vi "Log Error.vi"(8 "Error In":errorcluster, 10 "Error To Log":errorcluster, 11 "Error Handling In":refnum<class "Error Handling.lvclass">) -> (0 "Error Out":errorcluster, 3 "Error Handling Out":refnum<class "Error Handling.lvclass">)   [LabVIEW 2021, in "Error Handling.lvclass"]
uses:
  Error Handling.lvclass
  Accessors/Log File Reference/Get Log File Reference.vi
  Accessors/Log File Reference/Set Log File Reference.vi
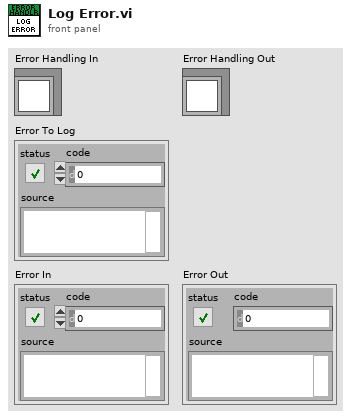
[diagram p1: front panel]
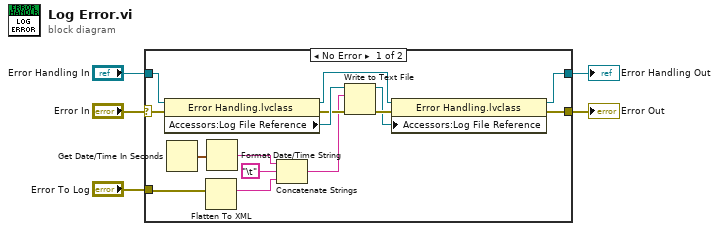
[diagram p0: block diagram]
diagram:
  n1 = case shown="No Error" "Error In" {
    selector: "Error In" -> [w20 w21]
    tunnel: "Error Handling In" -> [w19 w22]
    tunnel: [w12 w22] -> w3
    tunnel: [w15 w21] -> w2
    tunnel: "Error To Log" -> [w10 _]
    frame No Error {
      n2 = property class="Error Handling.lvclass"(reference=w19, error in=w20) -> (reference out=w14:refnum<class "Error Handling.lvclass">, error out=w17:errorcluster, "Accessors:Log File Reference"=w18:refnum<file>)
      n3 = Get Date/Time In Seconds() -> (seconds since 1Jan1904=w11:timestamp)
      n4 = Flatten To XML(6:w10) -> (2:w8:string)
      n5 = Format Date/Time String(seconds (now)=w11) -> (date/time string=w9:string)  [unwired: 2 in]
      n6 = Concatenate Strings(w9, "\t", w8) -> (w6:string)
      n7 = Write to Text File(file (use dialog)=w18, text=w6, error in=w17) -> (refnum out=w13:refnum<file>, error out=w16:errorcluster)  [unwired: 1 in, 1 out]
      n8 = property class="Error Handling.lvclass"(reference=w14, error in=w16, "Accessors:Log File Reference"=w13) -> (reference out=w12:refnum<class "Error Handling.lvclass">, error out=w15:errorcluster)
    }
    frame Error {
    }
  }
  "Error Handling Out" <- w3
  "Error Out" <- w2
